vi "Motor-Controls.vi"(6 "Downwards":i16, 7 "Still":i16, 8 "Upwards":i16) -> ()   [LabVIEW 2020]
uses:
  <userlib>/_NI I2C IP/FPGA/NI I2C IP FPGA.lvlib
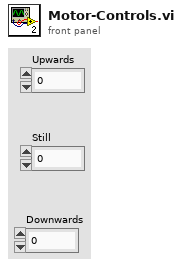
[diagram p1: front panel]
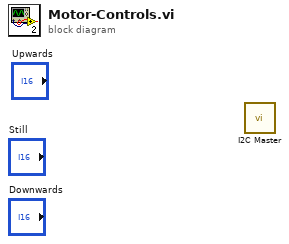
[diagram p0: block diagram]
diagram:
  n1 = call <userlib>:"I2C Master.vi"() -> ()  [unwired: 13 in, 3 out]
